vi "niDTS GNSS GPS Rx RF Test UTIL GNSS to GPS Results.vi"(1 "GNSS Results":T2) -> (0 "GPS Results":T1)   [LabVIEW 2014, in "niDTS GNSS.lvlib"]
uses:
  niDTS GNSS.lvlib
  RF Test/Includes/niDTS GNSS RF Test INC Results.ctl
  Includes/niDTS GNSS GPS Rx RF Test INC Results.ctl
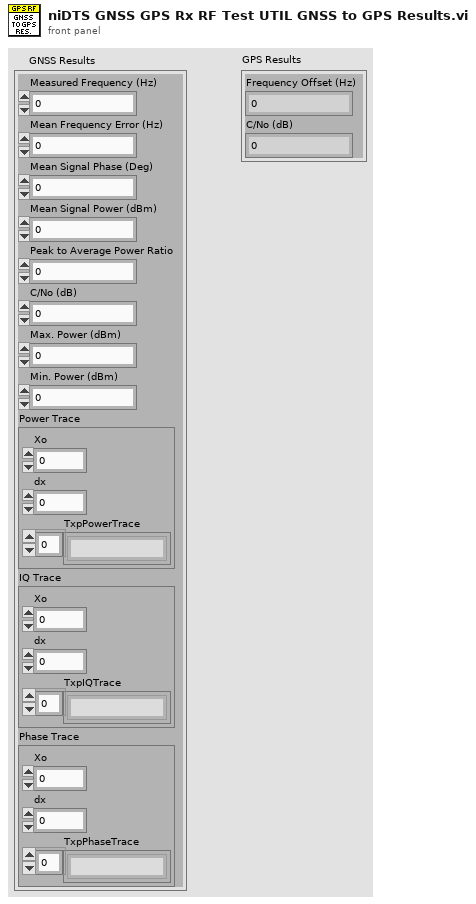
[diagram p1: front panel]
types:
  T1 = typedef "niDTS GNSS.lvlib/niDTS GNSS GPS Rx RF Test INC Results.ctl" = cluster{"Frequency Offset (Hz)":dbl, "C/No (dB)":dbl}
  T2 = typedef "niDTS GNSS.lvlib/niDTS GNSS RF Test INC Results.ctl" = cluster{"Measured Frequency (Hz)":dbl, "Mean Frequency Error (Hz)":dbl, "Mean Signal Phase (Deg)":dbl, "Mean Signal Power (dBm)":dbl, "Peak to Average Power Ratio":dbl, "C/No (dB)":dbl, "Max. Power (dBm)":dbl, "Min. Power (dBm)":dbl, "Power Trace":cluster{"Xo":dbl, "dx":dbl, "TxpPowerTrace":string[]}, "IQ Trace":cluster{"Xo":dbl, "dx":dbl, "TxpIQTrace":string[]}, "Phase Trace":cluster{"Xo":dbl, "dx":dbl, "TxpPhaseTrace":string[]}}
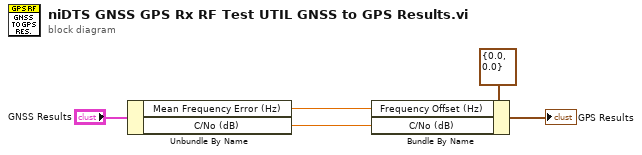
[diagram p0: block diagram]
diagram:
  n1 = Unbundle By Name("GNSS Results") -> ("Mean Frequency Error (Hz)"=w2:dbl, "C/No (dB)"=w1:dbl)
  n2 = Bundle By Name(cluster=T1 {"Frequency Offset (Hz)"=0.0, "C/No (dB)"=0.0} ("GPS Results"), "Frequency Offset (Hz)"=w2, "C/No (dB)"=w1) -> (→"GPS Results":T1)
